vi "Path 1.vi"() -> (3 "appended path":path)   [LabVIEW 2014]
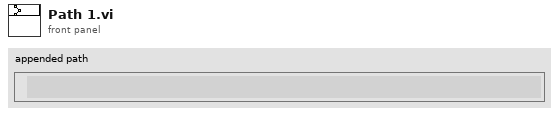
[diagram p1: front panel]
types:
  T1 = enum32{"invalid app kind", "Development System", "Run Time System", "Student Edition", "Embedded LabVIEW", "Evaluation", "Custom"}
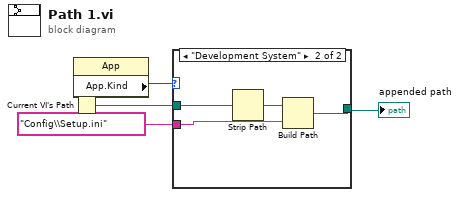
[diagram p0: block diagram]
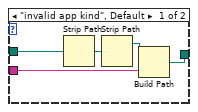
[diagram p2: hidden frame]
diagram:
  n1 = Current VI's Path() -> (path=w2:path)
  n2 = property class="App"() -> ("App.Kind"=w1:T1)  [unwired: 2 in, 2 out]
  n3 = case shown="\"Development System\"" w1 {
    tunnel: w2 -> [w9 w13]
    tunnel: "Config\\Setup.ini" -> [w7 w12]
    tunnel: [w6 w11] -> w4
    frame "invalid app kind", Default {
      n4 = Strip Path(path=w9) -> (stripped path=w5:path)  [unwired: 1 out]
      n5 = Strip Path(path=w5) -> (stripped path=w8:path)  [unwired: 1 out]
      n6 = Build Path(base path=w8, name or relative path=w7) -> (appended path=w6:path)
    }
    frame "Development System" {
      n7 = Strip Path(path=w13) -> (stripped path=w10:path)  [unwired: 1 out]
      n8 = Build Path(base path=w10, name or relative path=w12) -> (appended path=w11:path)
    }
  }
  "appended path" <- w4
